vi "Project.vi"() -> ()   [LabVIEW 2023]
uses:
  <vilib>/Instr/_visa.llb/VISA Configure Serial Port (Instr).vi
panel:
  out "Current Speed":dbl
  in  "Stop":bool
  in  "Speed":i32(knob) scale=0.0..9.0
  in  "Left":bool
  in  "Right":bool
  in  "Backward":bool
  in  "Forward":bool
  in  "Stop":bool
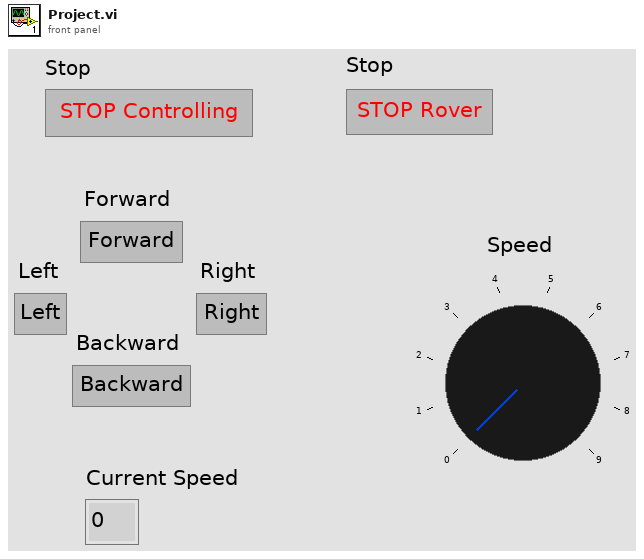
[diagram p1: front panel]
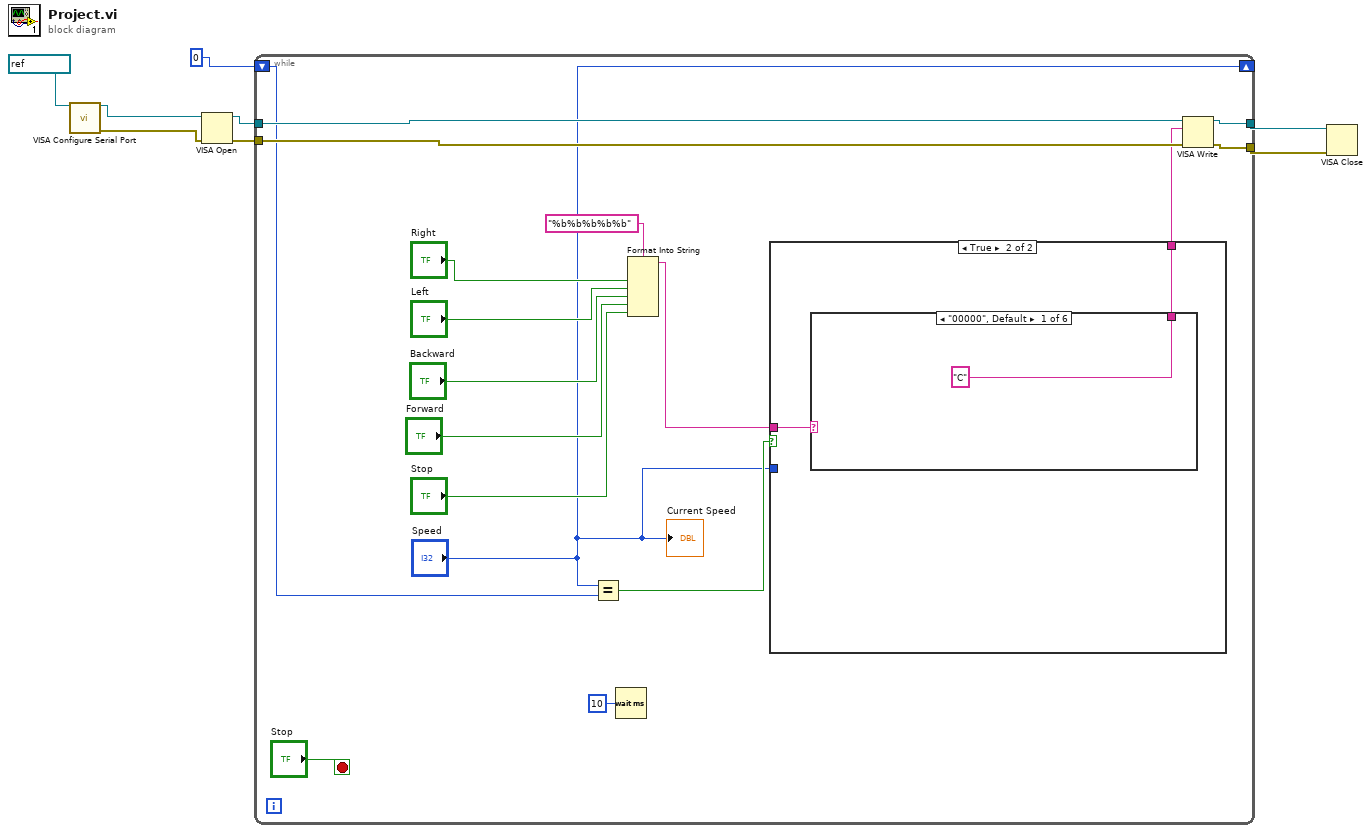
[diagram p0: block diagram]
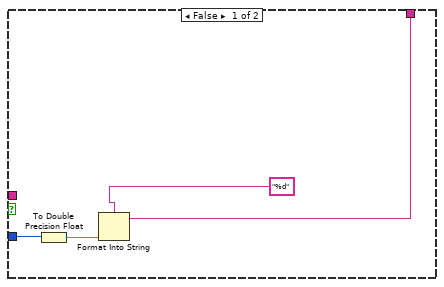
[diagram p2: hidden frame]
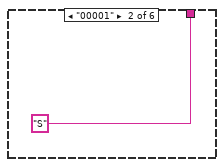
[diagram p3: hidden frame]
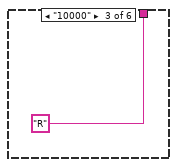
[diagram p4: hidden frame]
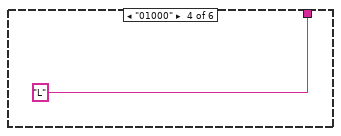
[diagram p5: hidden frame]
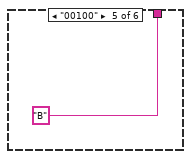
[diagram p6: hidden frame]
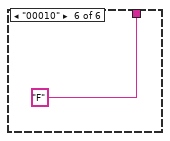
[diagram p7: hidden frame]
diagram:
  n1 = call-poly "VISA Configure Serial Port"("VISA resource name"=refnum<visa-resource-name> "COM5") -> ("VISA resource name out"=w2:refnum<visa-resource-name>, "error out"=w5:errorcluster)  [unwired: 13 in]
  n2 = VISA Open(error in (no error)=w5, VISA resource name=w2) -> (VISA resource name=w8:refnum<visa-resource-name>, error out=w6:errorcluster)  [unwired: 3 in]
  n3 = while {
    tunnel: w8 -> [w25]
    tunnel: [w23] -> w3
    tunnel: [w22] -> w7
    tunnel: w6 -> [w24]
    shift-right: ["Speed"] -> _
    shift-left: 0 -> [w20]
    stop <- "Stop" stop-if-true
    n4 = Equal?(x="Speed", y=w20) -> (x = y?=w10:bool)
    n5 = Wait (ms)(milliseconds to wait=u32 10) -> ()  [unwired: 1 out]
    n6 = Format Into String(format string="%b%b%b%b%b", "Right", "Left", "Backward", "Forward", "Stop") -> (resulting string=w13:string)  [unwired: 2 in, 1 out]
    n7 = case shown="True" w10 {
      tunnel: w13 -> [_ w31]
      tunnel: [w29 w30] -> w12
      tunnel: "Speed" -> [w27 _]
      frame False {
        n8 = To Double Precision Float(number=w27) -> (double precision float=w26:dbl)
        n9 = Format Into String(format string="%d", w26) -> (resulting string=w29:string)  [unwired: 2 in, 1 out]
      }
      frame True {
        n10 = case shown="\"00000\", Default" w31 {
          tunnel: ["C" "S" "R" "L" "B" "F"] -> w30
          frame "00000", Default {
          }
          frame "00001" {
          }
          frame "10000" {
          }
          frame "01000" {
          }
          frame "00100" {
          }
          frame "00010" {
          }
        }
      }
    }
    n11 = VISA Write(VISA resource name=w25, write buffer=w12, error in (no error)=w24) -> (VISA resource name out=w23:refnum<visa-resource-name>, error out=w22:errorcluster)  [unwired: 1 out]
    "Current Speed" <- "Speed"
  }
  n12 = VISA Close(VISA resource name=w3, error in (no error)=w7) -> ()  [unwired: 1 out]
